vi "Read NewTestRole.vi"(8 "error in (no error)":errorcluster, 11 "KeeperPlay in":refnum<class "KeeperPlay.lvclass">) -> (0 "error out":errorcluster, 2 "NewTestRole.lvclass":refnum<class "NewTestRole.lvclass">, 3 "KeeperPlay out":refnum<class "KeeperPlay.lvclass">)   [LabVIEW 2022 SP3, in "KeeperPlay.lvclass"]
uses:
  KeeperPlay.lvclass
  NewTestRole/NewTestRole.lvclass
  KeeperPlay.lvclass/KeeperPlay.ctl
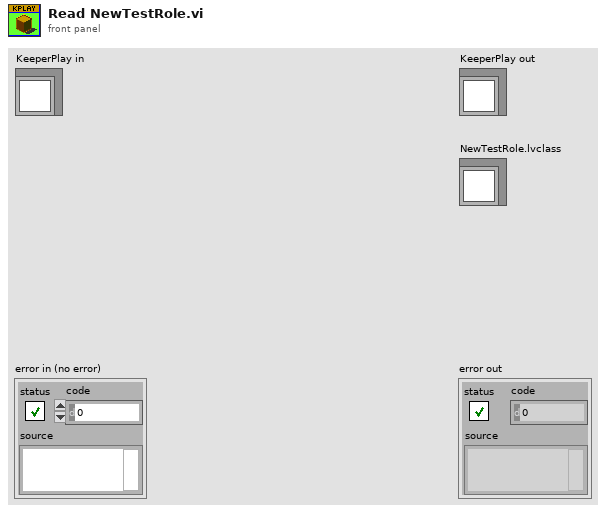
[diagram p1: front panel]
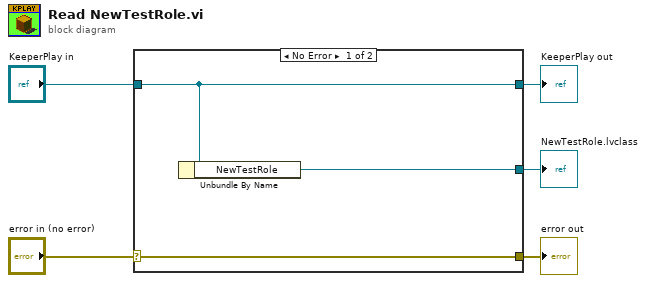
[diagram p0: block diagram]
diagram:
  n1 = case shown="No Error" "error in (no error)" {
    selector: "error in (no error)" -> [w8 w9]
    tunnel: [w8 w9] -> w4
    tunnel: [w7 w10] -> w2
    tunnel: "KeeperPlay in" -> [w7 w10]
    tunnel: [w6 _] -> w1
    frame No Error {
      n2 = Unbundle By Name(w7) -> ("NewTestRole"=w6:refnum<class "NewTestRole.lvclass">)
    }
    frame Error {
    }
  }
  "error out" <- w4
  "KeeperPlay out" <- w2
  "NewTestRole.lvclass" <- w1
